vi "result map.vi"(9 "output":dbl[](array[numeric])) -> (1 "note":string)   [LabVIEW 2016]
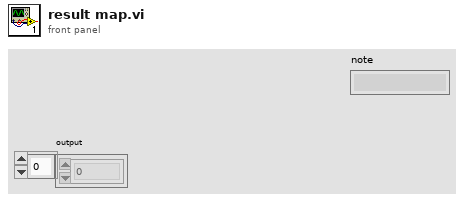
[diagram p1: front panel]
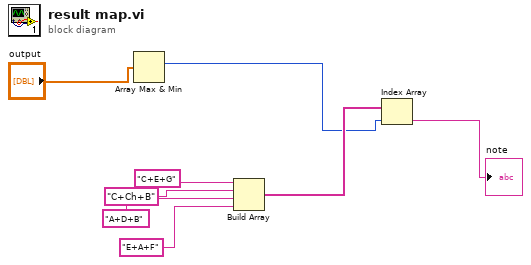
[diagram p0: block diagram]
diagram:
  n1 = Array Max & Min(array="output") -> (max index (indices)=w1:i32)  [unwired: 3 out]
  n2 = Build Array("C+E+G", "C+Ch+B", "A+D+B", "E+A+F") -> (w4:string[])
  n3 = Index Array(array=w4, index=w1) -> (element=→"note":string)
